vi "ExportMeas2TXT1.vi"(1 "File Path":path) -> (0 "error out 2":errorcluster)   [LabVIEW 2010]
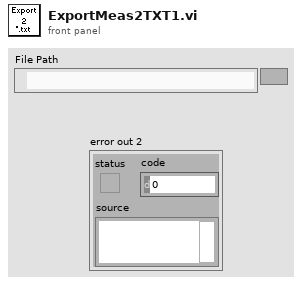
[diagram p1: front panel]
types:
  T1 = enum32{"existing file", "new file", "new or existing file", "existing dir", "new dir", "new or existing dir", "existing file (use LLBs)", "new file (use LLBs)", "new or existing file (use LLBs)", "new or existing file or directory (use LLBs)"}
  T2 = enum16{"open", "open or create", "create or replace", "create", "open (read only)"}
  T3 = cluster{"Array":string[], "MeasData":cluster{"Charge":i32, "U_Charge":i32[], "Shift":i32, "WinW":i32, "Qr":i32[][], "Ph":i32[][], "y_hist":i32[][], "x_hist":i32[][]}}[]
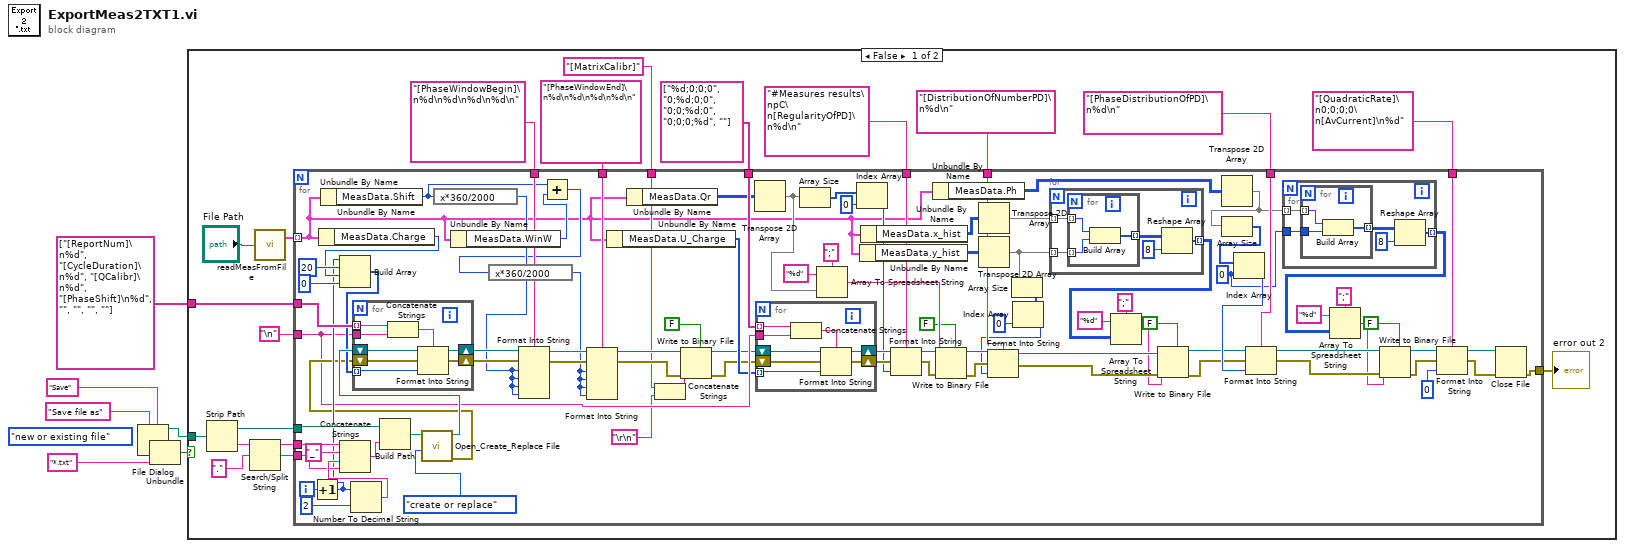
[diagram p0: block diagram]
diagram:
  (unwired) T1."new or existing file" ("select mode (2)")
  n1 = File Dialog(5:"Save" ("pattern"), 6:"*.txt" ("pattern"), 7:"Save file as" ("prompt")) -> (0:w1:errorcluster, 1:w5:bool, 3:w4:path)  [unwired: 4 in, 1 out]
  n2 = Unbundle(w1) -> ()  [unwired: 3 out]
  n3 = case shown="False" w5 {
    tunnel: w4 -> [w24 _]
    tunnel: string[] ["[ReportNum]\n%d", "[CycleDuration]\n%d", "[QCalibr]\n%d", "[PhaseShift]\n%d", "", "", "", ""] -> [w18 _]
    frame False {
      n4 = Strip Path(path=w24) -> (stripped path=w23:path, name=w22:string)
      n5 = Search/Split String(string=w22, search string/char (-)=".") -> (substring before match=w20:string, match + rest of string=w19:string)  [unwired: 1 in, 1 out]
      n6 = call "readMeasFromFile.vi"("path"="File Path") -> ("data"=w26:T3)  [unwired: 1 out]
      n7 = for {
        tunnel: w26 -> [w51] mode=indexing
        tunnel: w23 -> [w115]
        tunnel: w20 -> [w120]
        tunnel: w19 -> [w116]
        tunnel: w18 -> [w107]
        tunnel: "\n" -> [w89]
        tunnel: "[PhaseWindowBegin]\n%d\n%d\n%d\n%d\n" -> [w97]
        tunnel: [w100] -> w8
        tunnel: "[PhaseWindowEnd]\n%d\n%d\n%d\n%d\n" -> [w96]
        tunnel: string[] ["%d;0;0;0", "0;%d;0;0", "0;0;%d;0", "0;0;0;%d", ""] -> [w90]
        tunnel: "[MatrixCalibr]" -> [w83]
        tunnel: "#Measures results\npC\n[RegularityOfPD]\n%d\n" -> [w78]
        tunnel: "[DistributionOfNumberPD]\n%d\n" -> [w66]
        tunnel: "[PhaseDistributionOfPD]\n%d\n" -> [w45]
        tunnel: "[QuadraticRate]\n0;0;0;0\n[AvCurrent]\n%d" -> [w34]
        i -> [w112]
        w44 = 0 ("index")
        n8 = Increment(x=w112) -> (x+1=w104:i32)
        n9 = Unbundle By Name(w51) -> ("MeasData.Charge"=w110:i32)
        n10 = Unbundle By Name(w51) -> ("MeasData.Shift"=w94:i32)
        n11 = Build Array(w104, 20 ("element"), w110, 0 ("element")) -> (w106:i32[])
        n12 = Number To Decimal String(number=w104, width (-)=i16 2) -> (decimal integer string=w117:string)
        n13 = Concatenate Strings(w120, "_" ("string"), w117, w116) -> (w114:string)
        n14 = Build Path(base path=w115, name or relative path=w114) -> (appended path=w113:path)
        n15 = call <vilib>:"Open_Create_Replace File.vi"("function (open:0)"=T2."create or replace", "file path"=w113) -> ("error out"=w102:errorcluster, "refnum"=w108:refnum<file>)  [unwired: 6 in, 2 out]
        n16 = for {
          tunnel: w107 -> [w152] mode=indexing
          tunnel: w89 -> [w151]
          tunnel: w106 -> [w148] mode=indexing
          shift-right: [w147] -> w103
          shift-left: w108 -> [w149]
          shift-right: [w146] -> w101
          shift-left: w102 -> [w145]
          n17 = Concatenate Strings(w152, w151) -> (w150:string)
          n18 = Format Into String(format string=w150, initial string=w149, error in=w145, w148) -> (resulting string=w147:refnum<file>, error out=w146:errorcluster)
        }
        n19 = expression code="x*360/2000"(w94) -> (w95:i32)
        n20 = Unbundle By Name(w51) -> ("MeasData.WinW"=w93:i32)
        n21 = Format Into String(format string=w97, initial string=w103, error in=w101, w95, w95, w95, w95) -> (resulting string=w98:refnum<file>, error out=w99:errorcluster)
        n22 = Add(x=w94, y=w93) -> (x+y=w91:i32)
        n23 = expression code="x*360/2000"(w91) -> (w92:i32)
        n24 = Format Into String(format string=w96, initial string=w98, error in=w99, w92, w92, w92, w92) -> (resulting string=w87:refnum<file>, error out=w85:errorcluster)
        n25 = Unbundle By Name(w51) -> ("MeasData.U_Charge"=w88:i32[])
        n26 = Unbundle By Name(w51) -> ("MeasData.Qr"=w72:i32[][])
        n27 = Concatenate Strings(w83, "\r\n") -> (w81:string)
        n28 = Write to Binary File(file (use dialog)=w87, data=w81, error in=w85, 5:FALSE ("prepend array or string size? (T)")) -> (refnum out=w86:refnum<file>, error out=w84:errorcluster)  [unwired: 2 in, 1 out]
        n29 = Transpose 2D Array(2D array=w72) -> (transposed array=w68:i32[][])
        n30 = for {
          tunnel: w90 -> [w144] mode=indexing
          tunnel: w89 -> [w143]
          tunnel: w88 -> [w140] mode=indexing
          shift-right: [w139] -> w80
          shift-left: w86 -> [w141]
          shift-right: [w138] -> w79
          shift-left: w84 -> [w137]
          n31 = Concatenate Strings(w144, w143) -> (w142:string)
          n32 = Format Into String(format string=w142, initial string=w141, error in=w137, w140) -> (resulting string=w139:refnum<file>, error out=w138:errorcluster)
        }
        n33 = Array Size(array=w68) -> (size(s)=w77:i32[])
        n34 = Array To Spreadsheet String(delimiter (Tab)=";", array=w68, 3:"%d" ("format (%.3f)")) -> (spreadsheet string=w69:string)
        n35 = Index Array(array=w77, index=0) -> (element=w75:i32)
        n36 = Unbundle By Name(w51) -> ("MeasData.y_hist"=w63:i32[][])
        n37 = Unbundle By Name(w51) -> ("MeasData.x_hist"=w64:i32[][])
        n38 = Format Into String(format string=w78, initial string=w80, error in=w79, w75) -> (resulting string=w74:refnum<file>, error out=w73:errorcluster)
        n39 = Unbundle By Name(w51) -> ("MeasData.Ph"=w50:i32[][])
        n40 = Write to Binary File(file (use dialog)=w74, data=w69, error in=w73, 5:FALSE ("prepend array or string size? (T)")) -> (refnum out=w65:refnum<file>, error out=w67:errorcluster)  [unwired: 2 in, 1 out]
        n41 = Transpose 2D Array(2D array=w64) -> (transposed array=w62:i32[][])
        n42 = Transpose 2D Array(2D array=w63) -> (transposed array=w60:i32[][])
        n43 = Array Size(array=w60) -> (size(s)=w59:i32[])
        n44 = Index Array(array=w59, index=0) -> (element=w58:i32)
        n45 = Format Into String(format string=w66, initial string=w65, error in=w67, w58) -> (resulting string=w54:refnum<file>, error out=w53:errorcluster)
        n46 = for {
          tunnel: w62 -> [w133] mode=indexing
          tunnel: w60 -> [w132] mode=indexing
          tunnel: [w129] -> w55 mode=indexing
          n47 = for {
            tunnel: w133 -> [w136] mode=indexing
            tunnel: w132 -> [w135] mode=indexing
            tunnel: [w134] -> w131 mode=indexing
            n48 = Build Array(w136, w135) -> (w134:i32[])
          }
          n49 = Reshape Array(w131, 8 ("dimension size")) -> (w129:i32[])
        }
        n50 = Array To Spreadsheet String(delimiter (Tab)=";", array=w55, 3:"%d" ("format (%.3f)")) -> (spreadsheet string=w52:string)
        n51 = Write to Binary File(file (use dialog)=w54, data=w52, error in=w53, 5:FALSE ("prepend array or string size? (T)")) -> (refnum out=w46:refnum<file>, error out=w47:errorcluster)  [unwired: 2 in, 1 out]
        n52 = Transpose 2D Array(2D array=w50) -> (transposed array=w43:i32[][])
        n53 = Array Size(array=w43) -> (size(s)=w49:i32[])
        n54 = Index Array(array=w49, index=w44) -> (element=w48:i32)
        n55 = Format Into String(format string=w45, initial string=w46, error in=w47, w48) -> (resulting string=w39:refnum<file>, error out=w38:errorcluster)
        n56 = for {
          tunnel: w43 -> [w125] mode=indexing
          tunnel: [w122] -> w40 mode=indexing
          tunnel: w44 -> [w121]
          n57 = for {
            tunnel: w125 -> [w128] mode=indexing
            tunnel: [w127] -> w124 mode=indexing
            tunnel: w121 -> [w126]
            n58 = Build Array(w128, w126) -> (w127:i32[])
          }
          n59 = Reshape Array(w124, 8 ("dimension size")) -> (w122:i32[])
        }
        n60 = Array To Spreadsheet String(delimiter (Tab)=";", array=w40, 3:"%d" ("format (%.3f)")) -> (spreadsheet string=w37:string)
        n61 = Write to Binary File(file (use dialog)=w39, data=w37, error in=w38, 5:FALSE ("prepend array or string size? (T)")) -> (refnum out=w36:refnum<file>, error out=w33:errorcluster)  [unwired: 2 in, 1 out]
        n62 = Format Into String(format string=w34, initial string=w36, error in=w33, 0 ("input 1")) -> (resulting string=w35:refnum<file>, error out=w31:errorcluster)
        n63 = Close File(refnum=w35, error in=w31) -> (error out=w100:errorcluster)  [unwired: 1 out]
      }
      "error out 2" <- w8
    }
    frame True {
    }
  }
